vi "Build NIPKG.vi"(5 "Files Generated by Build":path[](array[path]), 6 "Top Level/Always Included VIs":path[](array[path]), 7 "Destination Path":path, 8 "error in (no error)":errorcluster, 9 "Target Name":string, 10 "Build Specification Name":string, 11 "Project Path":path) -> (0 "error out":errorcluster)   [LabVIEW 2016]
panel:
  in  "Maintainer":string="National Instruments"
  out "return code":i32
  out "standard input":string
  out "standard error":string
  out "standard output":string
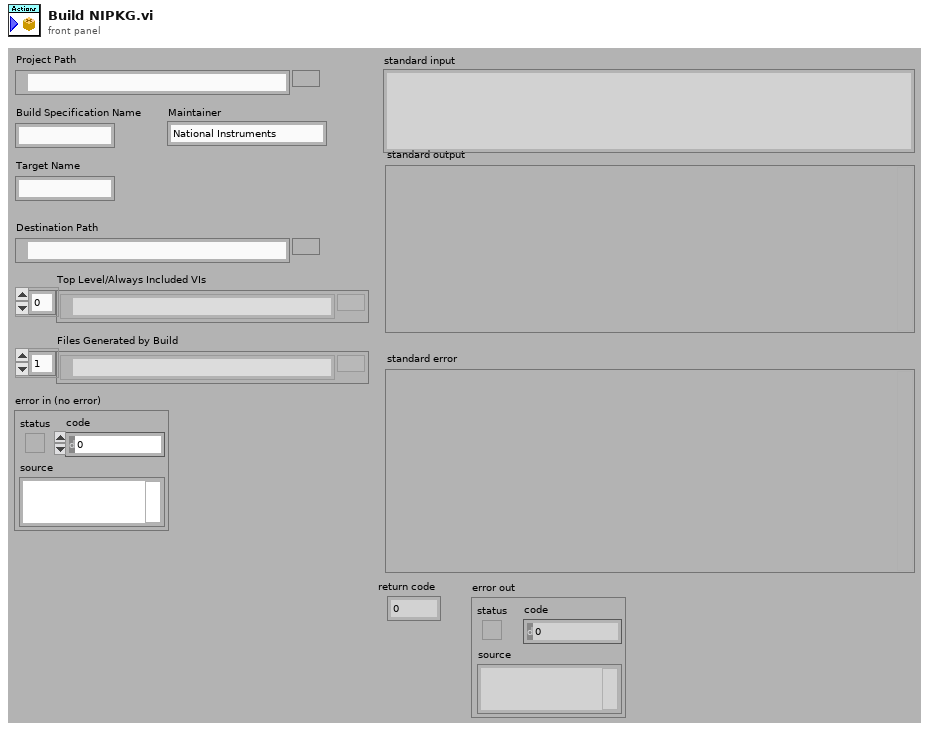
[diagram p1: front panel]
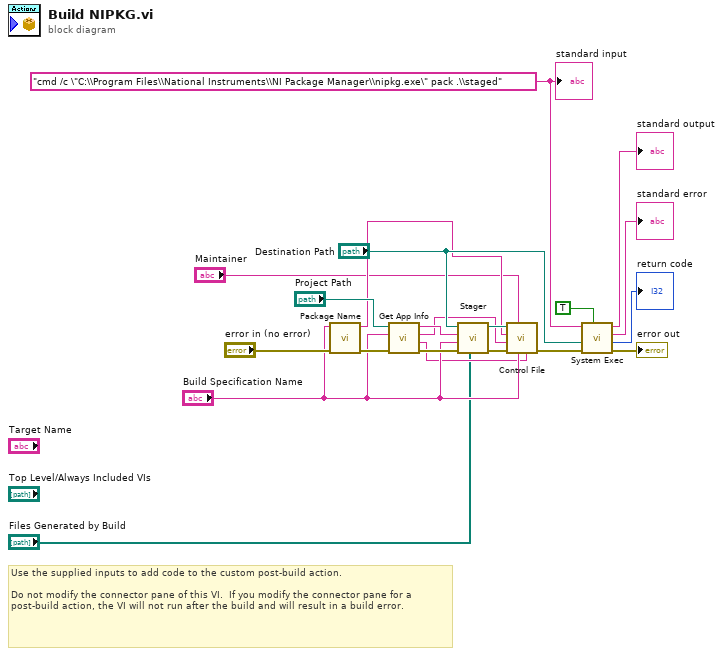
[diagram p0: block diagram]
diagram:
  w8 = "cmd /c \"C:\\Program Files\\National Instruments\\NI Package Manager\\nipkg.exe\" pack .\\staged" ("standard input")
  # "Use the supplied inputs to add code to the custom post-build action.\n\nDo not modify the connector pane of this VI.  If you modify the connector pane for a post-build action, the VI will not run after the build and will result in a build error."
  n1 = call "Package Name.vi"("error in (no error)"="error in (no error)", "Build Specification Name"="Build Specification Name") -> ("error out"=w13:errorcluster, "Package Name"=w6:string)  [unwired: 8 in]
  n2 = call "Get App Info.vi"("error in"=w13, "Build Spec Name"="Build Specification Name", "Project Path"="Project Path") -> ("error out"=w12:errorcluster, "Description"=w3:string, "Version"=w5:string, "Vendor"=w18:string)  [unwired: 4 in, 1 out]
  n3 = call "Stager.vi"("Files Generated by Build"="Files Generated by Build", "error in (no error)"=w12, "Product"="Build Specification Name", "Vendor"=w18, "Destination Path"="Destination Path") -> ("error out"=w11:errorcluster, "Staged Path"=w7:path)  [unwired: 5 in]
  n4 = call "Control File.vi"("Description"=w3, "Display Name"="Build Specification Name", "Maintainer"="Maintainer", "error in (no error)"=w11, "Version"=w5, "Package Name"=w6, "Stage Path"=w7) -> ("error out"=w10:errorcluster)  [unwired: 3 in, 1 out]
  n5 = call <vilib>:"System Exec.vi"("wait until completion? (T)"=TRUE, "error in (no error)"=w10, "working directory"="Destination Path", "command line"=w8) -> ("error out"=→"error out":errorcluster, "return code"=→"return code":i32, "standard error"=→"standard error":string, "standard output"=→"standard output":string)  [unwired: 4 in]
  "standard input" <- w8
